vi "SP_OEE_2_test.vi"() -> ()   [LabVIEW 2017] (continued)
                      tunnel: w15923 -> [w16181]
                      tunnel: w15922 -> [w16177]
                      tunnel: [w16176] -> w15907
                      tunnel: w15921 -> [w16176]
                      tunnel: w15920 -> [w16237]
                      tunnel: w15919 -> [w16230]
                      tunnel: w15918 -> [w16221]
                      tunnel: w15917 -> [w16229]
                      tunnel: w15916 -> [w16219]
                      tunnel: w15915 -> [w16228]
                      tunnel: w15914 -> [w16217]
                      tunnel: w15913 -> [w16227]
                      tunnel: w15912 -> [w16215]
                      tunnel: w15911 -> [w16251]
                      tunnel: w15910 -> [w16250]
                      tunnel: w15909 -> [w16226]
                      tunnel: w15908 -> [w16213]
                      tunnel: [w16251] -> w15906
                      tunnel: [w16250] -> w15905
                      tunnel: [w16244] -> w15904
                      tunnel: [w16237] -> w15903
                      tunnel: [w16236] -> w15902
                      tunnel: [w16235] -> w15901
                      tunnel: [w16234] -> w15900
                      tunnel: [w16233] -> w15899
                      tunnel: [w16232] -> w15898
                      tunnel: [w16231] -> w15897
                      tunnel: [w16230] -> w15896
                      tunnel: [w16229] -> w15895
                      tunnel: [w16228] -> w15894
                      tunnel: [w16227] -> w15893
                      tunnel: [w16226] -> w15892
                      tunnel: [w16211] -> w15891
                      tunnel: w15907 -> [w16211]
                      tunnel: [w16264] -> _
                      tunnel: [w16260] -> _
                      tunnel: w15906 -> [w16261]
                      tunnel: w15905 -> [w16264]
                      tunnel: w15904 -> [w16255]
                      tunnel: w15903 -> [w16262]
                      tunnel: w15902 -> [_]
                      tunnel: w15901 -> [_]
                      tunnel: w15900 -> [_]
                      tunnel: w15899 -> [w16252]
                      tunnel: w15898 -> [_]
                      tunnel: w15897 -> [w16256]
                      tunnel: w15896 -> [_]
                      tunnel: w15895 -> [_]
                      tunnel: w15894 -> [_]
                      tunnel: w15893 -> [w16253]
                      tunnel: w15892 -> [_]
                      tunnel: w15891 -> [w16259]
                      frame #0 {
                        w15995 = "%Y-%m-%d" ("time format string (%c)")
                        n2900 = Decimal String To Number(string=w15981) -> (number=w15982:i32)  [unwired: 2 in, 1 out]
                        n2901 = property on="Table" class="Tbl (strict)"("Visible"=TRUE) -> ()  [unwired: 2 in, 2 out]
                        n2902 = Format Date/Time String(time format string (%c)=w15995, seconds (now)=w15987) -> (date/time string=w15996:string)  [unwired: 1 in]
                        n2903 = Format Date/Time String(time format string (%c)=w15995, seconds (now)=w15986) -> (date/time string=w15994:string)  [unwired: 1 in]
                        n2904 = Format Into String(format string="Where BREAKDOWN_DATE between '%s' and '%s' and  SHIFT_ID = '%d'  ", w15996, w15994, w15982) -> (resulting string=w15993:string)  [unwired: 2 in, 1 out]
                        n2905 = call <vilib>:"DB Tools Select Data.vi"("condition"=w15993, "error in (no error)"=w16002, "columns"=string[] ["BREAKDOWN_DATE"], "table"="STATION_1_LOG_HISTORY", "connection reference"=w16004) -> ("error out"=w15989:errorcluster, "data"=w15992:variant[][], "connection reference out"=w16003:T2)  [unwired: 1 in]
                        n2906 = property on="Table 2" class="Tbl (strict)"("Visible"=FALSE) -> ()  [unwired: 2 in, 2 out]
                        n2907 = xnode "Database Variant To Data"("database variant"=w15992, "error in (no error)"=w15989, "type"=string[][] [] ("Elements Found")) -> ("data"=w15990:string[][], "error out"=w15988:errorcluster)
                        n2908 = Index Array(array=w15990, index (col)=0 ("disabled index (col)")) -> (element=w15998:string[])  [unwired: 1 in]
                        n2909 = call "Search_1d_array_element.vi"("Count in"=string[] [] ("Elements Found"), "BD Date"=w15998, "Elements Found in"=string[] [] ("Elements Found")) -> ("Elements Found out"=w15985:string[])  [unwired: 4 in, 2 out]
                        n2910 = Build Array(w15985) -> (w16008:string[][])
                        n2911 = Transpose 2D Array(2D array=w16008) -> (transposed array=w16007:string[][])
                      }
                      frame #1 {
                        n2912 = disable-structure shown="Enabled" {
                          disable-tunnel: w16070 -> [w16081 w16083]
                          disable-tunnel: [w16080 w16083] -> w16069
                          disable-tunnel: w16068 -> [w16079 w16084]
                          disable-tunnel: [w16078 w16084] -> w16067
                          disable-tunnel: w16065 -> [w16076 _]
                          disable-tunnel: w16064 -> [w16075 _]
                          disable-tunnel: [w16074 _] -> w16063
                          disable-tunnel: [w16073 _] -> w16060
                          disable-tunnel: w16058 -> [w16072 _]
                          disable-tunnel: w16055 -> [w16071 w16082]
                          disable-tunnel: [_ w16082] -> w16054
                          frame Disabled {
                            n2913 = call "Stack_holderwise_total_bd_count_&_duration_2.vi"("Refnum in"=w16081, "BREAKDOWN_STK_HOLD_ID"=1, "condition"=w16072, "Form Date"=w16076, "To Date"=w16075, "error in (no error)"=w16079, "Shift"=w16071) -> ("Refnum out"=w16080:T2, "Count out"=w16074:string[], "appended array"=w16073:dbl[], "error out"=w16078:errorcluster)  [unwired: 5 in]
                          }
                          frame Enabled {
                          }
                        }
                        n2914 = call "NUMERIC TO STRING.vi"("appended array"=w16060) -> ("Array"=w16059:string[])  [unwired: 4 in]
                        n2915 = call "Insert_empty_element_with_zero.vi"("searched date"=w16063, "fixed date"=w16061) -> ("O/P"=w16056:string[])  [unwired: 9 in]
                        n2916 = call "Insert_empty_element_with_zero.vi"("searched date"=w16059, "fixed date"=w16061) -> ("O/P"=w16062:string[])  [unwired: 9 in]
                      }
                      frame #2 {
                        n2917 = disable-structure shown="Enabled" {
                          disable-tunnel: w16100 -> [w16114 w16116]
                          disable-tunnel: [w16113 w16116] -> w16099
                          disable-tunnel: w16098 -> [w16112 w16117]
                          disable-tunnel: [w16111 w16117] -> w16097
                          disable-tunnel: w16096 -> [w16110 _]
                          disable-tunnel: w16095 -> [w16109 _]
                          disable-tunnel: [w16108 _] -> w16094
                          disable-tunnel: [w16107 _] -> w16090
                          disable-tunnel: w16088 -> [w16106 _]
                          disable-tunnel: w16086 -> [w16104 w16115]
                          disable-tunnel: [_ w16115] -> w16085
                          frame Disabled {
                            n2918 = call "Stack_holderwise_total_bd_count_&_duration_2.vi"("Refnum in"=w16112, "BREAKDOWN_STK_HOLD_ID"=2, "condition"=w16106, "Form Date"=w16110, "To Date"=w16109, "error in (no error)"=w16114, "Shift"=w16104) -> ("Refnum out"=w16111:T2, "Count out"=w16108:string[], "appended array"=w16107:dbl[], "error out"=w16113:errorcluster)  [unwired: 5 in]
                          }
                          frame Enabled {
                          }
                        }
                        n2919 = call "Insert_empty_element_with_zero.vi"("searched date"=w16094, "fixed date"=w16091) -> ("O/P"=w16093:string[])  [unwired: 9 in]
                        n2920 = call "NUMERIC TO STRING.vi"("appended array"=w16090) -> ("Array"=w16089:string[])  [unwired: 4 in]
                        n2921 = call "Insert_empty_element_with_zero.vi"("searched date"=w16089, "fixed date"=w16091) -> ("O/P"=w16092:string[])  [unwired: 9 in]
                      }
                      frame #3 {
                        n2922 = disable-structure shown="Enabled" {
                          disable-tunnel: w16133 -> [w16149 w16151]
                          disable-tunnel: [w16148 w16151] -> w16132
                          disable-tunnel: w16131 -> [w16147 w16152]
                          disable-tunnel: [w16146 w16152] -> w16130
                          disable-tunnel: w16129 -> [w16145 _]
                          disable-tunnel: w16128 -> [w16144 _]
                          disable-tunnel: [w16143 _] -> w16127
                          disable-tunnel: [w16142 _] -> w16123
                          disable-tunnel: w16121 -> [w16141 _]
                          disable-tunnel: w16119 -> [w16139 w16150]
                          disable-tunnel: [_ w16150] -> w16118
                          frame Disabled {
                            n2923 = call "Stack_holderwise_total_bd_count_&_duration_2.vi"("Refnum in"=w16147, "BREAKDOWN_STK_HOLD_ID"=3, "condition"=w16141, "Form Date"=w16145, "To Date"=w16144, "error in (no error)"=w16149, "Shift"=w16139) -> ("Refnum out"=w16146:T2, "Count out"=w16143:string[], "appended array"=w16142:dbl[], "error out"=w16148:errorcluster)  [unwired: 5 in]
                          }
                          frame Enabled {
                          }
                        }
                        n2924 = call "Insert_empty_element_with_zero.vi"("searched date"=w16127, "fixed date"=w16124) -> ("O/P"=w16126:string[])  [unwired: 9 in]
                        n2925 = call "NUMERIC TO STRING.vi"("appended array"=w16123) -> ("Array"=w16122:string[])  [unwired: 4 in]
                        n2926 = call "Insert_empty_element_with_zero.vi"("searched date"=w16122, "fixed date"=w16124) -> ("O/P"=w16125:string[])  [unwired: 9 in]
                      }
                      frame #4 {
                        n2927 = call "Stack_holderwise_total_bd_count_&_duration_2.vi"("Refnum in"=w16167, "BREAKDOWN_STK_HOLD_ID"=4, "condition"=w16156, "Form Date"=w16164, "To Date"=w16163, "error in (no error)"=w16168, "Shift"=w16153) -> ("Refnum out"=w16166:T2, "Count out"=w16162:string[], "appended array"=w16158:dbl[], "error out"=w16165:errorcluster)  [unwired: 5 in]
                        n2928 = call "Insert_empty_element_with_zero.vi"("searched date"=w16162, "fixed date"=w16159) -> ("O/P"=w16161:string[])  [unwired: 9 in]
                        n2929 = call "NUMERIC TO STRING.vi"("appended array"=w16158) -> ("Array"=w16157:string[])  [unwired: 4 in]
                        n2930 = call "Insert_empty_element_with_zero.vi"("searched date"=w16157, "fixed date"=w16159) -> ("O/P"=w16160:string[])  [unwired: 9 in]
                      }
                      frame #5 {
                        n2931 = disable-structure shown="Enabled" {
                          disable-tunnel: w16189 -> [w16207 w16210]
                          disable-tunnel: [w16206 w16210] -> w16188
                          disable-tunnel: w16187 -> [w16205 w16209]
                          disable-tunnel: [w16204 w16209] -> w16186
                          disable-tunnel: w16185 -> [w16203 _]
                          disable-tunnel: w16184 -> [w16202 _]
                          disable-tunnel: [w16201 _] -> w16183
                          disable-tunnel: [w16200 _] -> w16179
                          disable-tunnel: w16177 -> [w16199 _]
                          frame Disabled {
                            n2932 = call "Stack_holderwise_total_bd_count_&_duration.vi"("Refnum in"=w16205, "BREAKDOWN_STK_HOLD_ID"=5, "condition"=w16199, "Form Date"=w16202, "To Date"=w16203, "error in (no error)"=w16207) -> ("Refnum out"=w16204:T2, "Count out"=w16201:string[], "appended array"=w16200:dbl[], "error out"=w16206:errorcluster)  [unwired: 6 in]
                          }
                          frame Enabled {
                          }
                        }
                        n2933 = call "NUMERIC TO STRING.vi"("appended array"=w16179) -> ("Array"=w16178:string[])  [unwired: 4 in]
                        n2934 = call "Insert_empty_element_with_zero.vi"("searched date"=w16183, "fixed date"=w16181) -> ("O/P"=w16182:string[])  [unwired: 9 in]
                        n2935 = call "Insert_empty_element_with_zero.vi"("searched date"=w16178, "fixed date"=w16181) -> ("O/P"=w16180:string[])  [unwired: 9 in]
                      }
                      frame #6 {
                        n2936 = call "String to numeric.vi"("Array"=w16221) -> ("Array 2"=w16220:dbl[])  [unwired: 4 in]
                        n2937 = call "String to numeric.vi"("Array"=w16219) -> ("Array 2"=w16218:dbl[])  [unwired: 4 in]
                        n2938 = call "String to numeric.vi"("Array"=w16217) -> ("Array 2"=w16216:dbl[])  [unwired: 4 in]
                        n2939 = call "String to numeric.vi"("Array"=w16215) -> ("Array 2"=w16214:dbl[])  [unwired: 4 in]
                        n2940 = call "String to numeric.vi"("Array"=w16213) -> ("Array 2"=w16212:dbl[])  [unwired: 4 in]
                        n2941 = Decimal String To Number(string=w16226) -> (number=w16245:i32[])  [unwired: 2 in, 1 out]
                        n2942 = Decimal String To Number(string=w16227) -> (number=w16246:i32[])  [unwired: 2 in, 1 out]
                        n2943 = Decimal String To Number(string=w16228) -> (number=w16247:i32[])  [unwired: 2 in, 1 out]
                        n2944 = Decimal String To Number(string=w16229) -> (number=w16248:i32[])  [unwired: 2 in, 1 out]
                        n2945 = Decimal String To Number(string=w16230) -> (number=w16243:i32[])  [unwired: 2 in, 1 out]
                        n2946 = Compound Arithmetic op=ADD(w16220, w16218, w16216, w16214, w16212) -> (w16223:dbl[])
                        n2947 = Build Array(w16221) -> (w16242:string[][])
                        n2948 = Build Array(w16219) -> (w16241:string[][])
                        n2949 = Build Array(w16217) -> (w16240:string[][])
                        n2950 = Build Array(w16215) -> (w16239:string[][])
                        n2951 = Build Array(w16213) -> (w16238:string[][])
                        n2952 = Number To Fractional String(number=w16223, precision (6)=i16 2) -> (F-format string=w16222:string[])  [unwired: 2 in]
                        n2953 = Compound Arithmetic op=ADD(w16245, w16246, w16247, w16248, w16243) -> (w16249:i32[])
                        n2954 = Transpose 2D Array(2D array=w16242) -> (transposed array=w16236:string[][])
                        n2955 = Transpose 2D Array(2D array=w16241) -> (transposed array=w16235:string[][])
                        n2956 = Transpose 2D Array(2D array=w16240) -> (transposed array=w16234:string[][])
                        n2957 = Transpose 2D Array(2D array=w16239) -> (transposed array=w16233:string[][])
                        n2958 = Transpose 2D Array(2D array=w16238) -> (transposed array=w16232:string[][])
                        n2959 = Number To Decimal String(number=w16249) -> (decimal integer string=w16244:string[])  [unwired: 1 in]
                        n2960 = Build Array(w16222) -> (w16225:string[][])
                        n2961 = Transpose 2D Array(2D array=w16225) -> (transposed array=w16231:string[][])
                      }
                      frame #7 {
                        w16254 = string[] [""]
                        n2962 = Insert Into Array(array=w16262, index (col)=1 ("disabled index (col)"), new element #1=w16254, new element #2=w16254, new element #3=w16254, new element #4=w16254, new element #5=w16254, new element #6=w16254, new element #7=w16253, new element #8=w16252, new element #9=w16254, new element #10=w16254, new element #11=w16255, new element #12=w16256) -> (w16258:string[][])  [unwired: 1 in]
                        n2963 = call "flot graph for month n year.vi"("BD Date"=w16259, "error in (no error)"=w16261, "Count total"=w16255) -> ("error out"=w16260:errorcluster, "Run-Time Status"=w16257:cluster{"Array 2":timestamp[], dbl[]})  [unwired: 7 in]
                        n2964 = local write "Run-Time Status"(w16257) -> ()
                        n2965 = local write "Table"(w16258) -> ()
                      }
                    }
                  }
                  frame "3" {
                    n2966 = flat-sequence {
                      tunnel: w16274 -> [w16388]
                      tunnel: w16273 -> [w16386]
                      tunnel: [w16372] -> w16364
                      tunnel: [w16387] -> w16363
                      tunnel: w16272 -> [_]
                      tunnel: [w16391] -> w16362
                      tunnel: [w16371] -> w16361
                      tunnel: [w16370] -> w16360
                      tunnel: [w16369] -> w16359
                      tunnel: w16271 -> [w16371]
                      tunnel: w16270 -> [w16370]
                      tunnel: ["Where BREAKDOWN_DATE between '%s'and '%s' and BREAKDOWN_STK_HOLD_ID ='%d' and  SHIFT_ID = '%d' "] -> w16358
                      tunnel: [w16369] -> w16357
                      tunnel: w16269 -> [w16365]
                      tunnel: [w16365] -> w16268
                      tunnel: w16364 -> [w16452]
                      tunnel: w16363 -> [w16454]
                      tunnel: w16362 -> [w16450]
                      tunnel: w16361 -> [w16449]
                      tunnel: w16360 -> [w16448]
                      tunnel: [w16451] -> w16356
                      tunnel: [w16453] -> w16355
                      tunnel: [w16450] -> w16354
                      tunnel: [w16440] -> w16353
                      tunnel: [w16446] -> w16352
                      tunnel: [w16449] -> w16351
                      tunnel: [w16448] -> w16350
                      tunnel: w16359 -> [w16445]
                      tunnel: [w16445] -> w16349
                      tunnel: w16358 -> [w16442]
                      tunnel: [w16442] -> w16348
                      tunnel: [w16441] -> w16347
                      tunnel: w16357 -> [w16441]
                      tunnel: w16268 -> [w16439]
                      tunnel: [w16438] -> w16267
                      tunnel: w16356 -> [w16484]
                      tunnel: w16355 -> [w16482]
                      tunnel: w16354 -> [w16487]
                      tunnel: w16353 -> [w16486]
                      tunnel: w16352 -> [w16485]
                      tunnel: w16351 -> [w16480]
                      tunnel: w16350 -> [w16479]
                      tunnel: [w16487] -> w16346
                      tunnel: [w16486] -> w16345
                      tunnel: [w16485] -> w16344
                      tunnel: [w16483] -> w16343
                      tunnel: [w16477] -> w16342
                      tunnel: [w16476] -> w16341
                      tunnel: [w16481] -> w16340
                      tunnel: [w16480] -> w16339
                      tunnel: [w16479] -> w16338
                      tunnel: w16349 -> [w16475]
                      tunnel: [w16475] -> w16337
                      tunnel: w16348 -> [w16472]
                      tunnel: [w16472] -> w16336
                      tunnel: [w16471] -> w16335
                      tunnel: w16347 -> [w16471]
                      tunnel: w16267 -> [w16470]
                      tunnel: [w16469] -> w16266
                      tunnel: w16346 -> [w16522]
                      tunnel: w16345 -> [w16521]
                      tunnel: w16344 -> [w16520]
                      tunnel: w16343 -> [w16517]
                      tunnel: w16342 -> [w16519]
                      tunnel: w16341 -> [w16518]
                      tunnel: w16340 -> [w16515]
                      tunnel: w16339 -> [w16513]
                      tunnel: w16338 -> [w16512]
                      tunnel: [w16522] -> w16334
                      tunnel: [w16521] -> w16333
                      tunnel: [w16520] -> w16332
                      tunnel: [w16519] -> w16331
                      tunnel: [w16518] -> w16330
                      tunnel: [w16516] -> w16329
                      tunnel: [w16510] -> w16328
                      tunnel: [w16509] -> w16327
                      tunnel: [w16514] -> w16326
                      tunnel: [w16513] -> w16325
                      tunnel: [w16512] -> w16324
                      tunnel: w16337 -> [w16508]
                      tunnel: [w16508] -> w16323
                      tunnel: w16336 -> [w16505]
                      tunnel: [w16505] -> w16322
                      tunnel: [w16504] -> w16321
                      tunnel: w16335 -> [w16504]
                      tunnel: w16266 -> [w16503]
                      tunnel: [w16502] -> w16265
                      tunnel: w16334 -> [w16559]
                      tunnel: w16333 -> [w16558]
                      tunnel: w16332 -> [w16557]
                      tunnel: w16331 -> [w16556]
                      tunnel: w16330 -> [w16555]
                      tunnel: w16329 -> [w16552]
                      tunnel: w16328 -> [w16554]
                      tunnel: w16327 -> [w16553]
                      tunnel: w16326 -> [w16551]
                      tunnel: w16325 -> [w16548]
                      tunnel: w16324 -> [w16547]
                      tunnel: [w16559] -> w16320
                      tunnel: [w16558] -> w16319
                      tunnel: [w16557] -> w16318
                      tunnel: [w16556] -> w16317
                      tunnel: [w16555] -> w16316
                      tunnel: [w16554] -> w16315
                      tunnel: [w16553] -> w16314
                      tunnel: [w16550] -> w16313
                      tunnel: [w16549] -> w16312
                      tunnel: [w16545] -> w16311
                      tunnel: [w16544] -> w16310
                      tunnel: [w16548] -> w16309
                      tunnel: [w16547] -> w16308
                      tunnel: w16323 -> [w16543]
                      tunnel: [w16543] -> w16307
                      tunnel: w16322 -> [w16540]
                      tunnel: [w16540] -> w16306
                      tunnel: [w16539] -> w16305
                      tunnel: w16321 -> [w16539]
                      tunnel: w16265 -> [w16537]
                      tunnel: w16320 -> [w16582]
                      tunnel: w16319 -> [w16581]
                      tunnel: w16318 -> [w16580]
                      tunnel: w16317 -> [w16579]
                      tunnel: w16316 -> [w16578]
                      tunnel: w16315 -> [w16577]
                      tunnel: w16314 -> [w16576]
                      tunnel: w16313 -> [w16571]
                      tunnel: w16312 -> [w16573]
                      tunnel: w16311 -> [w16575]
                      tunnel: w16310 -> [w16574]
                      tunnel: w16309 -> [w16568]
                      tunnel: w16308 -> [w16569]
                      tunnel: [w16582] -> w16304
                      tunnel: [w16581] -> w16303
                      tunnel: [w16580] -> w16302
                      tunnel: [w16579] -> w16301
                      tunnel: [w16578] -> w16300
                      tunnel: [w16577] -> w16299
                      tunnel: [w16576] -> w16298
                      tunnel: [w16575] -> w16297
                      tunnel: [w16574] -> w16296
                      tunnel: [w16572] -> w16295
                      tunnel: [w16570] -> w16294
                      tunnel: [w16566] -> w16293
                      tunnel: [w16564] -> w16292
                      tunnel: w16307 -> [w16565]
                      tunnel: w16306 -> [w16561]
                      tunnel: [w16560] -> w16291
                      tunnel: w16305 -> [w16560]
                      tunnel: w16304 -> [w16621]
                      tunnel: w16303 -> [w16614]
                      tunnel: w16302 -> [w16605]
                      tunnel: w16301 -> [w16613]
                      tunnel: w16300 -> [w16603]
                      tunnel: w16299 -> [w16612]
                      tunnel: w16298 -> [w16601]
                      tunnel: w16297 -> [w16611]
                      tunnel: w16296 -> [w16599]
                      tunnel: w16295 -> [w16635]
                      tunnel: w16294 -> [w16634]
                      tunnel: w16293 -> [w16610]
                      tunnel: w16292 -> [w16597]
                      tunnel: [w16635] -> w16290
                      tunnel: [w16634] -> w16289
                      tunnel: [w16628] -> w16288
                      tunnel: [w16621] -> w16287
                      tunnel: [w16620] -> w16286
                      tunnel: [w16619] -> w16285
                      tunnel: [w16618] -> w16284
                      tunnel: [w16617] -> w16283
                      tunnel: [w16616] -> w16282
                      tunnel: [w16615] -> w16281
                      tunnel: [w16614] -> w16280
                      tunnel: [w16613] -> w16279
                      tunnel: [w16612] -> w16278
                      tunnel: [w16611] -> w16277
                      tunnel: [w16610] -> w16276
                      tunnel: [w16595] -> w16275
                      tunnel: w16291 -> [w16595]
                      tunnel: [w16648] -> _
                      tunnel: [w16644] -> _
                      tunnel: w16290 -> [w16645]
                      tunnel: w16289 -> [w16648]
                      tunnel: w16288 -> [w16639]
                      tunnel: w16287 -> [w16646]
                      tunnel: w16286 -> [_]
                      tunnel: w16285 -> [_]
                      tunnel: w16284 -> [_]
                      tunnel: w16283 -> [w16636]
                      tunnel: w16282 -> [_]
                      tunnel: w16281 -> [w16640]
                      tunnel: w16280 -> [_]
                      tunnel: w16279 -> [_]
                      tunnel: w16278 -> [_]
                      tunnel: w16277 -> [w16637]
                      tunnel: w16276 -> [_]
                      tunnel: w16275 -> [w16643]
                      frame #0 {
                        w16379 = "%Y-%m-%d" ("time format string (%c)")
                        n2967 = Decimal String To Number(string=w16365) -> (number=w16366:i32)  [unwired: 2 in, 1 out]
                        n2968 = property on="Table" class="Tbl (strict)"("Visible"=TRUE) -> ()  [unwired: 2 in, 2 out]
                        n2969 = Format Date/Time String(time format string (%c)=w16379, seconds (now)=w16371) -> (date/time string=w16380:string)  [unwired: 1 in]
                        n2970 = Format Date/Time String(time format string (%c)=w16379, seconds (now)=w16370) -> (date/time string=w16378:string)  [unwired: 1 in]
                        n2971 = Format Into String(format string="Where BREAKDOWN_DATE between '%s' and '%s' and  SHIFT_ID = '%d'  ", w16380, w16378, w16366) -> (resulting string=w16377:string)  [unwired: 2 in, 1 out]
                        n2972 = call <vilib>:"DB Tools Select Data.vi"("condition"=w16377, "error in (no error)"=w16386, "columns"=string[] ["BREAKDOWN_DATE"], "table"="STATION_1_LOG_HISTORY", "connection reference"=w16388) -> ("error out"=w16373:errorcluster, "data"=w16376:variant[][], "connection reference out"=w16387:T2)  [unwired: 1 in]
                        n2973 = property on="Table 2" class="Tbl (strict)"("Visible"=FALSE) -> ()  [unwired: 2 in, 2 out]
                        n2974 = xnode "Database Variant To Data"("database variant"=w16376, "error in (no error)"=w16373, "type"=string[][] [] ("Elements Found")) -> ("data"=w16374:string[][], "error out"=w16372:errorcluster)
                        n2975 = Index Array(array=w16374, index (col)=0 ("disabled index (col)")) -> (element=w16382:string[])  [unwired: 1 in]
                        n2976 = call "Search_1d_array_element.vi"("Count in"=string[] [] ("Elements Found"), "BD Date"=w16382, "Elements Found in"=string[] [] ("Elements Found")) -> ("Elements Found out"=w16369:string[])  [unwired: 4 in, 2 out]
                        n2977 = Build Array(w16369) -> (w16392:string[][])
                        n2978 = Transpose 2D Array(2D array=w16392) -> (transposed array=w16391:string[][])
                      }
                      frame #1 {
                        n2979 = disable-structure shown="Enabled" {
                          disable-tunnel: w16454 -> [w16465 w16467]
                          disable-tunnel: [w16464 w16467] -> w16453
                          disable-tunnel: w16452 -> [w16463 w16468]
                          disable-tunnel: [w16462 w16468] -> w16451
                          disable-tunnel: w16449 -> [w16460 _]
                          disable-tunnel: w16448 -> [w16459 _]
                          disable-tunnel: [w16458 _] -> w16447
                          disable-tunnel: [w16457 _] -> w16444
                          disable-tunnel: w16442 -> [w16456 _]
                          disable-tunnel: w16439 -> [w16455 w16466]
                          disable-tunnel: [_ w16466] -> w16438
                          frame Disabled {
                            n2980 = call "Stack_holderwise_total_bd_count_&_duration_2.vi"("Refnum in"=w16465, "BREAKDOWN_STK_HOLD_ID"=1, "condition"=w16456, "Form Date"=w16460, "To Date"=w16459, "error in (no error)"=w16463, "Shift"=w16455) -> ("Refnum out"=w16464:T2, "Count out"=w16458:string[], "appended array"=w16457:dbl[], "error out"=w16462:errorcluster)  [unwired: 5 in]
                          }
                          frame Enabled {
                          }
                        }
                        n2981 = call "NUMERIC TO STRING.vi"("appended array"=w16444) -> ("Array"=w16443:string[])  [unwired: 4 in]
                        n2982 = call "Insert_empty_element_with_zero.vi"("searched date"=w16447, "fixed date"=w16445) -> ("O/P"=w16440:string[])  [unwired: 9 in]
                        n2983 = call "Insert_empty_element_with_zero.vi"("searched date"=w16443, "fixed date"=w16445) -> ("O/P"=w16446:string[])  [unwired: 9 in]
                      }
                      frame #2 {
                        n2984 = disable-structure shown="Enabled" {
                          disable-tunnel: w16484 -> [w16498 w16500]
                          disable-tunnel: [w16497 w16500] -> w16483
                          disable-tunnel: w16482 -> [w16496 w16501]
                          disable-tunnel: [w16495 w16501] -> w16481
                          disable-tunnel: w16480 -> [w16494 _]
                          disable-tunnel: w16479 -> [w16493 _]
                          disable-tunnel: [w16492 _] -> w16478
                          disable-tunnel: [w16491 _] -> w16474
                          disable-tunnel: w16472 -> [w16490 _]
                          disable-tunnel: w16470 -> [w16488 w16499]
                          disable-tunnel: [_ w16499] -> w16469
                          frame Disabled {
                            n2985 = call "Stack_holderwise_total_bd_count_&_duration_2.vi"("Refnum in"=w16496, "BREAKDOWN_STK_HOLD_ID"=2, "condition"=w16490, "Form Date"=w16494, "To Date"=w16493, "error in (no error)"=w16498, "Shift"=w16488) -> ("Refnum out"=w16495:T2, "Count out"=w16492:string[], "appended array"=w16491:dbl[], "error out"=w16497:errorcluster)  [unwired: 5 in]
                          }
                          frame Enabled {
                          }
                        }
                        n2986 = call "Insert_empty_element_with_zero.vi"("searched date"=w16478, "fixed date"=w16475) -> ("O/P"=w16477:string[])  [unwired: 9 in]
                        n2987 = call "NUMERIC TO STRING.vi"("appended array"=w16474) -> ("Array"=w16473:string[])  [unwired: 4 in]
                        n2988 = call "Insert_empty_element_with_zero.vi"("searched date"=w16473, "fixed date"=w16475) -> ("O/P"=w16476:string[])  [unwired: 9 in]
                      }
                      frame #3 {
                        n2989 = disable-structure shown="Enabled" {
                          disable-tunnel: w16517 -> [w16533 w16535]
                          disable-tunnel: [w16532 w16535] -> w16516
                          disable-tunnel: w16515 -> [w16531 w16536]
                          disable-tunnel: [w16530 w16536] -> w16514
                          disable-tunnel: w16513 -> [w16529 _]
                          disable-tunnel: w16512 -> [w16528 _]
                          disable-tunnel: [w16527 _] -> w16511
                          disable-tunnel: [w16526 _] -> w16507
                          disable-tunnel: w16505 -> [w16525 _]
                          disable-tunnel: w16503 -> [w16523 w16534]
                          disable-tunnel: [_ w16534] -> w16502
                          frame Disabled {
                            n2990 = call "Stack_holderwise_total_bd_count_&_duration_2.vi"("Refnum in"=w16531, "BREAKDOWN_STK_HOLD_ID"=3, "condition"=w16525, "Form Date"=w16529, "To Date"=w16528, "error in (no error)"=w16533, "Shift"=w16523) -> ("Refnum out"=w16530:T2, "Count out"=w16527:string[], "appended array"=w16526:dbl[], "error out"=w16532:errorcluster)  [unwired: 5 in]
                          }
                          frame Enabled {
                          }
                        }
                        n2991 = call "Insert_empty_element_with_zero.vi"("searched date"=w16511, "fixed date"=w16508) -> ("O/P"=w16510:string[])  [unwired: 9 in]
                        n2992 = call "NUMERIC TO STRING.vi"("appended array"=w16507) -> ("Array"=w16506:string[])  [unwired: 4 in]
                        n2993 = call "Insert_empty_element_with_zero.vi"("searched date"=w16506, "fixed date"=w16508) -> ("O/P"=w16509:string[])  [unwired: 9 in]
                      }
                      frame #4 {
                        n2994 = call "Stack_holderwise_total_bd_count_&_duration_2.vi"("Refnum in"=w16551, "BREAKDOWN_STK_HOLD_ID"=4, "condition"=w16540, "Form Date"=w16548, "To Date"=w16547, "error in (no error)"=w16552, "Shift"=w16537) -> ("Refnum out"=w16550:T2, "Count out"=w16546:string[], "appended array"=w16542:dbl[], "error out"=w16549:errorcluster)  [unwired: 5 in]
                        n2995 = call "Insert_empty_element_with_zero.vi"("searched date"=w16546, "fixed date"=w16543) -> ("O/P"=w16545:string[])  [unwired: 9 in]
                        n2996 = call "NUMERIC TO STRING.vi"("appended array"=w16542) -> ("Array"=w16541:string[])  [unwired: 4 in]
                        n2997 = call "Insert_empty_element_with_zero.vi"("searched date"=w16541, "fixed date"=w16543) -> ("O/P"=w16544:string[])  [unwired: 9 in]
                      }
                      frame #5 {
                        n2998 = disable-structure shown="Enabled" {
                          disable-tunnel: w16573 -> [w16591 w16594]
                          disable-tunnel: [w16590 w16594] -> w16572
                          disable-tunnel: w16571 -> [w16589 w16593]
                          disable-tunnel: [w16588 w16593] -> w16570
                          disable-tunnel: w16569 -> [w16587 _]
                          disable-tunnel: w16568 -> [w16586 _]
                          disable-tunnel: [w16585 _] -> w16567
                          disable-tunnel: [w16584 _] -> w16563
                          disable-tunnel: w16561 -> [w16583 _]
                          frame Disabled {
                            n2999 = call "Stack_holderwise_total_bd_count_&_duration.vi"("Refnum in"=w16589, "BREAKDOWN_STK_HOLD_ID"=5, "condition"=w16583, "Form Date"=w16586, "To Date"=w16587, "error in (no error)"=w16591) -> ("Refnum out"=w16588:T2, "Count out"=w16585:string[], "appended array"=w16584:dbl[], "error out"=w16590:errorcluster)  [unwired: 6 in]
                          }
                          frame Enabled {
                          }
                        }
                        n3000 = call "NUMERIC TO STRING.vi"("appended array"=w16563) -> ("Array"=w16562:string[])  [unwired: 4 in]
                        n3001 = call "Insert_empty_element_with_zero.vi"("searched date"=w16567, "fixed date"=w16565) -> ("O/P"=w16566:string[])  [unwired: 9 in]
                        n3002 = call "Insert_empty_element_with_zero.vi"("searched date"=w16562, "fixed date"=w16565) -> ("O/P"=w16564:string[])  [unwired: 9 in]
                      }
                      frame #6 {
                        n3003 = call "String to numeric.vi"("Array"=w16605) -> ("Array 2"=w16604:dbl[])  [unwired: 4 in]
                        n3004 = call "String to numeric.vi"("Array"=w16603) -> ("Array 2"=w16602:dbl[])  [unwired: 4 in]
                        n3005 = call "String to numeric.vi"("Array"=w16601) -> ("Array 2"=w16600:dbl[])  [unwired: 4 in]
                        n3006 = call "String to numeric.vi"("Array"=w16599) -> ("Array 2"=w16598:dbl[])  [unwired: 4 in]
                        n3007 = call "String to numeric.vi"("Array"=w16597) -> ("Array 2"=w16596:dbl[])  [unwired: 4 in]
                        n3008 = Decimal String To Number(string=w16610) -> (number=w16629:i32[])  [unwired: 2 in, 1 out]
                        n3009 = Decimal String To Number(string=w16611) -> (number=w16630:i32[])  [unwired: 2 in, 1 out]
                        n3010 = Decimal String To Number(string=w16612) -> (number=w16631:i32[])  [unwired: 2 in, 1 out]
                        n3011 = Decimal String To Number(string=w16613) -> (number=w16632:i32[])  [unwired: 2 in, 1 out]
                        n3012 = Decimal String To Number(string=w16614) -> (number=w16627:i32[])  [unwired: 2 in, 1 out]
                        n3013 = Compound Arithmetic op=ADD(w16604, w16602, w16600, w16598, w16596) -> (w16607:dbl[])
                        n3014 = Build Array(w16605) -> (w16626:string[][])
                        n3015 = Build Array(w16603) -> (w16625:string[][])
                        n3016 = Build Array(w16601) -> (w16624:string[][])
                        n3017 = Build Array(w16599) -> (w16623:string[][])
                        n3018 = Build Array(w16597) -> (w16622:string[][])
                        n3019 = Number To Fractional String(number=w16607, precision (6)=i16 2) -> (F-format string=w16606:string[])  [unwired: 2 in]
                        n3020 = Compound Arithmetic op=ADD(w16629, w16630, w16631, w16632, w16627) -> (w16633:i32[])
                        n3021 = Transpose 2D Array(2D array=w16626) -> (transposed array=w16620:string[][])
                        n3022 = Transpose 2D Array(2D array=w16625) -> (transposed array=w16619:string[][])
                        n3023 = Transpose 2D Array(2D array=w16624) -> (transposed array=w16618:string[][])
                        n3024 = Transpose 2D Array(2D array=w16623) -> (transposed array=w16617:string[][])
                        n3025 = Transpose 2D Array(2D array=w16622) -> (transposed array=w16616:string[][])
                        n3026 = Number To Decimal String(number=w16633) -> (decimal integer string=w16628:string[])  [unwired: 1 in]
                        n3027 = Build Array(w16606) -> (w16609:string[][])
                        n3028 = Transpose 2D Array(2D array=w16609) -> (transposed array=w16615:string[][])
                      }
                      frame #7 {
                        w16638 = string[] [""]
                        n3029 = Insert Into Array(array=w16646, index (col)=1 ("disabled index (col)"), new element #1=w16638, new element #2=w16638, new element #3=w16638, new element #4=w16638, new element #5=w16638, new element #6=w16638, new element #7=w16637, new element #8=w16636, new element #9=w16638, new element #10=w16638, new element #11=w16639, new element #12=w16640) -> (w16642:string[][])  [unwired: 1 in]
                        n3030 = call "flot graph for month n year.vi"("BD Date"=w16643, "error in (no error)"=w16645, "Count total"=w16639) -> ("error out"=w16644:errorcluster, "Run-Time Status"=w16641:cluster{"Array 2":timestamp[], dbl[]})  [unwired: 7 in]
                        n3031 = local write "Run-Time Status"(w16641) -> ()
                        n3032 = local write "Table"(w16642) -> ()
                      }
                    }
                  }
                  frame "all" {
                  }
                }
              }
              frame "Production" {
                n3033 = local read "Shift"() -> (w16649:string)
                n3034 = case shown="\"1\"" w16649 {
                  selector: w16649 -> [_ w17024 w17413 w17802 _]
                  tunnel: w16654 -> [w16659 w17029 w17418 w17807 _]
                  tunnel: w16653 -> [w16658 w17028 w17417 w17806 _]
                  tunnel: w16652 -> [w16657 w17027 w17416 w17805 _]
                  tunnel: w16651 -> [w16656 w17026 w17415 w17804 _]
                  tunnel: w16650 -> [w16655 w17025 w17414 w17803 _]
                  frame "ALL", Default {
                    n3035 = flat-sequence {
                      tunnel: w16659 -> [w16771]
                      tunnel: w16658 -> [w16769]
                      tunnel: [w16755] -> w16749
                      tunnel: [w16770] -> w16748
                      tunnel: w16657 -> [_]
                      tunnel: [w16774] -> w16747
                      tunnel: [w16754] -> w16746
                      tunnel: [w16753] -> w16745
                      tunnel: [w16751] -> w16744
                      tunnel: w16656 -> [w16754]
                      tunnel: w16655 -> [w16753]
                      tunnel: ["Where BREAKDOWN_DATE between '%s'and '%s' and BREAKDOWN_STK_HOLD_ID ='%d'  "] -> w16743
                      tunnel: [w16751] -> w16742
                      tunnel: w16749 -> [w16833]
                      tunnel: w16748 -> [w16835]
                      tunnel: w16747 -> [w16831]
                      tunnel: w16746 -> [w16830]
                      tunnel: w16745 -> [w16829]
                      tunnel: [w16832] -> w16741
                      tunnel: [w16834] -> w16740
                      tunnel: [w16831] -> w16739
                      tunnel: [w16821] -> w16738
                      tunnel: [w16827] -> w16737
                      tunnel: [w16830] -> w16736
                      tunnel: [w16829] -> w16735
                      tunnel: w16744 -> [w16826]
                      tunnel: [w16826] -> w16734
                      tunnel: w16743 -> [w16823]
                      tunnel: [w16823] -> w16733
                      tunnel: [w16822] -> w16732
                      tunnel: w16742 -> [w16822]
                      tunnel: w16741 -> [w16861]
                      tunnel: w16740 -> [w16859]
                      tunnel: w16739 -> [w16864]
                      tunnel: w16738 -> [w16863]
                      tunnel: w16737 -> [w16862]
                      tunnel: w16736 -> [w16857]
                      tunnel: w16735 -> [w16856]
                      tunnel: [w16864] -> w16731
                      tunnel: [w16863] -> w16730
                      tunnel: [w16862] -> w16729
                      tunnel: [w16860] -> w16728
                      tunnel: [w16854] -> w16727
                      tunnel: [w16853] -> w16726
                      tunnel: [w16858] -> w16725
                      tunnel: [w16857] -> w16724
                      tunnel: [w16856] -> w16723
                      tunnel: w16734 -> [w16852]
                      tunnel: [w16852] -> w16722
                      tunnel: w16733 -> [w16849]
                      tunnel: [w16849] -> w16721
                      tunnel: [w16848] -> w16720
                      tunnel: w16732 -> [w16848]
                      tunnel: w16731 -> [w16895]
                      tunnel: w16730 -> [w16894]
                      tunnel: w16729 -> [w16893]
                      tunnel: w16728 -> [w16890]
                      tunnel: w16727 -> [w16892]
                      tunnel: w16726 -> [w16891]
                      tunnel: w16725 -> [w16888]
                      tunnel: w16724 -> [w16886]
                      tunnel: w16723 -> [w16885]
                      tunnel: [w16895] -> w16719
                      tunnel: [w16894] -> w16718
                      tunnel: [w16893] -> w16717
                      tunnel: [w16892] -> w16716
                      tunnel: [w16891] -> w16715
                      tunnel: [w16889] -> w16714
                      tunnel: [w16883] -> w16713
                      tunnel: [w16882] -> w16712
                      tunnel: [w16887] -> w16711
                      tunnel: [w16886] -> w16710
                      tunnel: [w16885] -> w16709
                      tunnel: w16722 -> [w16881]
                      tunnel: [w16881] -> w16708
                      tunnel: w16721 -> [w16878]
                      tunnel: [w16878] -> w16707
                      tunnel: [w16877] -> w16706
                      tunnel: w16720 -> [w16877]
                      tunnel: w16719 -> [w16928]
                      tunnel: w16718 -> [w16927]
                      tunnel: w16717 -> [w16926]
                      tunnel: w16716 -> [w16925]
                      tunnel: w16715 -> [w16924]
                      tunnel: w16714 -> [w16921]
                      tunnel: w16713 -> [w16923]
                      tunnel: w16712 -> [w16922]
                      tunnel: w16711 -> [w16920]
                      tunnel: w16710 -> [w16917]
                      tunnel: w16709 -> [w16916]
                      tunnel: [w16928] -> w16705
                      tunnel: [w16927] -> w16704
                      tunnel: [w16926] -> w16703
                      tunnel: [w16925] -> w16702
                      tunnel: [w16924] -> w16701
                      tunnel: [w16923] -> w16700
                      tunnel: [w16922] -> w16699
                      tunnel: [w16919] -> w16698
                      tunnel: [w16918] -> w16697
                      tunnel: [w16914] -> w16696
                      tunnel: [w16913] -> w16695
                      tunnel: [w16917] -> w16694
                      tunnel: [w16916] -> w16693
                      tunnel: w16708 -> [w16912]
                      tunnel: [w16912] -> w16692
                      tunnel: w16707 -> [w16909]
                      tunnel: [w16909] -> w16691
                      tunnel: [w16908] -> w16690
                      tunnel: w16706 -> [w16908]
                      tunnel: w16705 -> [w16964]
                      tunnel: w16704 -> [w16963]
                      tunnel: w16703 -> [w16962]
                      tunnel: w16702 -> [w16961]
                      tunnel: w16701 -> [w16960]
                      tunnel: w16700 -> [w16959]
                      tunnel: w16699 -> [w16958]
                      tunnel: w16698 -> [w16953]
                      tunnel: w16697 -> [w16955]
                      tunnel: w16696 -> [w16957]
                      tunnel: w16695 -> [w16956]
                      tunnel: w16694 -> [w16950]
                      tunnel: w16693 -> [w16951]
                      tunnel: [w16964] -> w16689
                      tunnel: [w16963] -> w16688
                      tunnel: [w16962] -> w16687
                      tunnel: [w16961] -> w16686
                      tunnel: [w16960] -> w16685
                      tunnel: [w16959] -> w16684
                      tunnel: [w16958] -> w16683
                      tunnel: [w16957] -> w16682
                      tunnel: [w16956] -> w16681
                      tunnel: [w16954] -> w16680
                      tunnel: [w16952] -> w16679
                      tunnel: [w16948] -> w16678
                      tunnel: [w16946] -> w16677
                      tunnel: w16692 -> [w16947]
                      tunnel: w16691 -> [w16943]
                      tunnel: [w16942] -> w16676
                      tunnel: w16690 -> [w16942]
                      tunnel: w16689 -> [w16991]
                      tunnel: w16688 -> [w16984]
                      tunnel: w16687 -> [w16975]
                      tunnel: w16686 -> [w16983]
                      tunnel: w16685 -> [w16973]
                      tunnel: w16684 -> [w16982]
                      tunnel: w16683 -> [w16971]
                      tunnel: w16682 -> [w16981]
                      tunnel: w16681 -> [w16969]
                      tunnel: w16680 -> [w17005]
                      tunnel: w16679 -> [w17004]
                      tunnel: w16678 -> [w16980]
                      tunnel: w16677 -> [w16967]
                      tunnel: [w17005] -> w16675
                      tunnel: [w17004] -> w16674
                      tunnel: [w16998] -> w16673
                      tunnel: [w16991] -> w16672
                      tunnel: [w16990] -> w16671
                      tunnel: [w16989] -> w16670
                      tunnel: [w16988] -> w16669
                      tunnel: [w16987] -> w16668
                      tunnel: [w16986] -> w16667
                      tunnel: [w16985] -> w16666
                      tunnel: [w16984] -> w16665
                      tunnel: [w16983] -> w16664
                      tunnel: [w16982] -> w16663
                      tunnel: [w16981] -> w16662
                      tunnel: [w16980] -> w16661
                      tunnel: [w16965] -> w16660
                      tunnel: w16676 -> [w16965]
                      tunnel: [w17018] -> _
                      tunnel: [w17014] -> _
                      tunnel: w16675 -> [w17015]
                      tunnel: w16674 -> [w17018]
                      tunnel: w16673 -> [w17009]
                      tunnel: w16672 -> [w17016]
                      tunnel: w16671 -> [_]
                      tunnel: w16670 -> [_]
                      tunnel: w16669 -> [_]
                      tunnel: w16668 -> [_]
                      tunnel: w16667 -> [w17008]
                      tunnel: w16666 -> [w17010]
                      tunnel: w16665 -> [_]
                      tunnel: w16664 -> [_]
                      tunnel: w16663 -> [_]
                      tunnel: w16662 -> [_]
                      tunnel: w16661 -> [w17007]
                      tunnel: w16660 -> [w17013]
                      frame #0 {
                        w16762 = "%Y-%m-%d" ("time format string (%c)")
                        n3036 = property on="Table" class="Tbl (strict)"("Visible"=TRUE) -> ()  [unwired: 2 in, 2 out]
                        n3037 = Format Date/Time String(time format string (%c)=w16762, seconds (now)=w16754) -> (date/time string=w16763:string)  [unwired: 1 in]
                        n3038 = Format Date/Time String(time format string (%c)=w16762, seconds (now)=w16753) -> (date/time string=w16761:string)  [unwired: 1 in]
                        n3039 = Format Into String(format string="Where BREAKDOWN_DATE between '%s' and '%s' ", w16763, w16761) -> (resulting string=w16760:string)  [unwired: 2 in, 1 out]
                        n3040 = call <vilib>:"DB Tools Select Data.vi"("condition"=w16760, "error in (no error)"=w16769, "columns"=string[] ["BREAKDOWN_DATE"], "table"="STATION_1_LOG_HISTORY", "connection reference"=w16771) -> ("error out"=w16756:errorcluster, "data"=w16759:variant[][], "connection reference out"=w16770:T2)  [unwired: 1 in]
                        n3041 = property on="Table 2" class="Tbl (strict)"("Visible"=FALSE) -> ()  [unwired: 2 in, 2 out]
                        n3042 = xnode "Database Variant To Data"("database variant"=w16759, "error in (no error)"=w16756, "type"=string[][] [] ("Elements Found")) -> ("data"=w16757:string[][], "error out"=w16755:errorcluster)
                        n3043 = Index Array(array=w16757, index (col)=0 ("disabled index (col)")) -> (element=w16765:string[])  [unwired: 1 in]
                        n3044 = call "Search_1d_array_element.vi"("Count in"=string[] [] ("Elements Found"), "BD Date"=w16765, "Elements Found in"=string[] [] ("Elements Found")) -> ("Elements Found out"=w16751:string[])  [unwired: 4 in, 2 out]
                        n3045 = Build Array(w16751) -> (w16775:string[][])
                        n3046 = Transpose 2D Array(2D array=w16775) -> (transposed array=w16774:string[][])
                      }
                      frame #1 {
                        n3047 = disable-structure shown="Enabled" {
                          disable-tunnel: w16835 -> [w16845 w16846]
                          disable-tunnel: [w16844 w16846] -> w16834
                          disable-tunnel: w16833 -> [w16843 w16847]
                          disable-tunnel: [w16842 w16847] -> w16832
                          disable-tunnel: w16830 -> [w16840 _]
                          disable-tunnel: w16829 -> [w16839 _]
                          disable-tunnel: [w16838 _] -> w16828
                          disable-tunnel: [w16837 _] -> w16825
                          disable-tunnel: w16823 -> [w16836 _]
                          frame Disabled {
                            n3048 = call "Stack_holderwise_total_bd_count_&_duration.vi"("Refnum in"=w16845, "BREAKDOWN_STK_HOLD_ID"=1, "condition"=w16836, "Form Date"=w16840, "To Date"=w16839, "error in (no error)"=w16843) -> ("Refnum out"=w16844:T2, "Count out"=w16838:string[], "appended array"=w16837:dbl[], "error out"=w16842:errorcluster)  [unwired: 6 in]
                          }
                          frame Enabled {
                          }
                        }
                        n3049 = call "NUMERIC TO STRING.vi"("appended array"=w16825) -> ("Array"=w16824:string[])  [unwired: 4 in]
                        n3050 = call "Insert_empty_element_with_zero.vi"("searched date"=w16828, "fixed date"=w16826) -> ("O/P"=w16821:string[])  [unwired: 9 in]
                        n3051 = call "Insert_empty_element_with_zero.vi"("searched date"=w16824, "fixed date"=w16826) -> ("O/P"=w16827:string[])  [unwired: 9 in]
                      }
                      frame #2 {
                        n3052 = disable-structure shown="Enabled" {
                          disable-tunnel: w16861 -> [w16874 w16876]
                          disable-tunnel: [w16873 w16876] -> w16860
                          disable-tunnel: w16859 -> [w16872 w16875]
                          disable-tunnel: [w16871 w16875] -> w16858
                          disable-tunnel: w16857 -> [w16870 _]
                          disable-tunnel: w16856 -> [w16869 _]
                          disable-tunnel: [w16868 _] -> w16855
                          disable-tunnel: [w16867 _] -> w16851
                          disable-tunnel: w16849 -> [w16866 _]
                          frame Disabled {
                            n3053 = call "Stack_holderwise_total_bd_count_&_duration.vi"("Refnum in"=w16872, "BREAKDOWN_STK_HOLD_ID"=2, "condition"=w16866, "Form Date"=w16870, "To Date"=w16869, "error in (no error)"=w16874) -> ("Refnum out"=w16871:T2, "Count out"=w16868:string[], "appended array"=w16867:dbl[], "error out"=w16873:errorcluster)  [unwired: 6 in]
                          }
                          frame Enabled {
                          }
                        }
                        n3054 = call "Insert_empty_element_with_zero.vi"("searched date"=w16855, "fixed date"=w16852) -> ("O/P"=w16854:string[])  [unwired: 9 in]
                        n3055 = call "NUMERIC TO STRING.vi"("appended array"=w16851) -> ("Array"=w16850:string[])  [unwired: 4 in]
                        n3056 = call "Insert_empty_element_with_zero.vi"("searched date"=w16850, "fixed date"=w16852) -> ("O/P"=w16853:string[])  [unwired: 9 in]
                      }
                      frame #3 {
                        n3057 = disable-structure shown="Enabled" {
                          disable-tunnel: w16890 -> [w16905 w16907]
                          disable-tunnel: [w16904 w16907] -> w16889
                          disable-tunnel: w16888 -> [w16903 w16906]
                          disable-tunnel: [w16902 w16906] -> w16887
                          disable-tunnel: w16886 -> [w16901 _]
                          disable-tunnel: w16885 -> [w16900 _]
                          disable-tunnel: [w16899 _] -> w16884
                          disable-tunnel: [w16898 _] -> w16880
                          disable-tunnel: w16878 -> [w16897 _]
                          frame Disabled {
                            n3058 = call "Stack_holderwise_total_bd_count_&_duration.vi"("Refnum in"=w16903, "BREAKDOWN_STK_HOLD_ID"=3, "condition"=w16897, "Form Date"=w16901, "To Date"=w16900, "error in (no error)"=w16905) -> ("Refnum out"=w16902:T2, "Count out"=w16899:string[], "appended array"=w16898:dbl[], "error out"=w16904:errorcluster)  [unwired: 6 in]
                          }
                          frame Enabled {
                          }
                        }
                        n3059 = call "Insert_empty_element_with_zero.vi"("searched date"=w16884, "fixed date"=w16881) -> ("O/P"=w16883:string[])  [unwired: 9 in]
                        n3060 = call "NUMERIC TO STRING.vi"("appended array"=w16880) -> ("Array"=w16879:string[])  [unwired: 4 in]
                        n3061 = call "Insert_empty_element_with_zero.vi"("searched date"=w16879, "fixed date"=w16881) -> ("O/P"=w16882:string[])  [unwired: 9 in]
                      }
                      frame #4 {
                        n3062 = disable-structure shown="Enabled" {
                          disable-tunnel: w16921 -> [w16938 w16940]
                          disable-tunnel: w16920 -> [w16937 w16939]
                          disable-tunnel: [w16936 w16939] -> w16919
                          disable-tunnel: [w16935 w16940] -> w16918
                          disable-tunnel: w16917 -> [w16934 _]
                          disable-tunnel: w16916 -> [w16933 _]
                          disable-tunnel: [w16932 _] -> w16915
                          disable-tunnel: [w16931 _] -> w16911
                          disable-tunnel: w16909 -> [w16930 _]
                          frame Disabled {
                            n3063 = call "Stack_holderwise_total_bd_count_&_duration.vi"("Refnum in"=w16937, "BREAKDOWN_STK_HOLD_ID"=4, "condition"=w16930, "Form Date"=w16934, "To Date"=w16933, "error in (no error)"=w16938) -> ("Refnum out"=w16936:T2, "Count out"=w16932:string[], "appended array"=w16931:dbl[], "error out"=w16935:errorcluster)  [unwired: 6 in]
                          }
                          frame Enabled {
                          }
                        }
                        n3064 = call "Insert_empty_element_with_zero.vi"("searched date"=w16915, "fixed date"=w16912) -> ("O/P"=w16914:string[])  [unwired: 9 in]
                        n3065 = call "NUMERIC TO STRING.vi"("appended array"=w16911) -> ("Array"=w16910:string[])  [unwired: 4 in]
                        n3066 = call "Insert_empty_element_with_zero.vi"("searched date"=w16910, "fixed date"=w16912) -> ("O/P"=w16913:string[])  [unwired: 9 in]
                      }
                      frame #5 {
                        n3067 = call "Stack_holderwise_total_bd_count_&_duration.vi"("Refnum in"=w16953, "BREAKDOWN_STK_HOLD_ID"=5, "condition"=w16943, "Form Date"=w16950, "To Date"=w16951, "error in (no error)"=w16955) -> ("Refnum out"=w16952:T2, "Count out"=w16949:string[], "appended array"=w16945:dbl[], "error out"=w16954:errorcluster)  [unwired: 6 in]
                        n3068 = call "NUMERIC TO STRING.vi"("appended array"=w16945) -> ("Array"=w16944:string[])  [unwired: 4 in]
                        n3069 = call "Insert_empty_element_with_zero.vi"("searched date"=w16949, "fixed date"=w16947) -> ("O/P"=w16948:string[])  [unwired: 9 in]
                        n3070 = call "Insert_empty_element_with_zero.vi"("searched date"=w16944, "fixed date"=w16947) -> ("O/P"=w16946:string[])  [unwired: 9 in]
                      }
                      frame #6 {
                        n3071 = call "String to numeric.vi"("Array"=w16975) -> ("Array 2"=w16974:dbl[])  [unwired: 4 in]
                        n3072 = call "String to numeric.vi"("Array"=w16973) -> ("Array 2"=w16972:dbl[])  [unwired: 4 in]
                        n3073 = call "String to numeric.vi"("Array"=w16971) -> ("Array 2"=w16970:dbl[])  [unwired: 4 in]
                        n3074 = call "String to numeric.vi"("Array"=w16969) -> ("Array 2"=w16968:dbl[])  [unwired: 4 in]
                        n3075 = call "String to numeric.vi"("Array"=w16967) -> ("Array 2"=w16966:dbl[])  [unwired: 4 in]
                        n3076 = Decimal String To Number(string=w16980) -> (number=w16999:i32[])  [unwired: 2 in, 1 out]
                        n3077 = Decimal String To Number(string=w16981) -> (number=w17000:i32[])  [unwired: 2 in, 1 out]
                        n3078 = Decimal String To Number(string=w16982) -> (number=w17001:i32[])  [unwired: 2 in, 1 out]
                        n3079 = Decimal String To Number(string=w16983) -> (number=w17002:i32[])  [unwired: 2 in, 1 out]
                        n3080 = Decimal String To Number(string=w16984) -> (number=w16997:i32[])  [unwired: 2 in, 1 out]
                        n3081 = Compound Arithmetic op=ADD(w16974, w16972, w16970, w16968, w16966) -> (w16977:dbl[])
                        n3082 = Build Array(w16975) -> (w16996:string[][])
                        n3083 = Build Array(w16973) -> (w16995:string[][])
                        n3084 = Build Array(w16971) -> (w16994:string[][])
                        n3085 = Build Array(w16969) -> (w16993:string[][])
                        n3086 = Build Array(w16967) -> (w16992:string[][])
                        n3087 = Number To Fractional String(number=w16977, precision (6)=i16 2) -> (F-format string=w16976:string[])  [unwired: 2 in]
                        n3088 = Compound Arithmetic op=ADD(w16999, w17000, w17001, w17002, w16997) -> (w17003:i32[])
                        n3089 = Transpose 2D Array(2D array=w16996) -> (transposed array=w16990:string[][])
                        n3090 = Transpose 2D Array(2D array=w16995) -> (transposed array=w16989:string[][])
                        n3091 = Transpose 2D Array(2D array=w16994) -> (transposed array=w16988:string[][])
                        n3092 = Transpose 2D Array(2D array=w16993) -> (transposed array=w16987:string[][])
                        n3093 = Transpose 2D Array(2D array=w16992) -> (transposed array=w16986:string[][])
                        n3094 = Number To Decimal String(number=w17003) -> (decimal integer string=w16998:string[])  [unwired: 1 in]
                        n3095 = Build Array(w16976) -> (w16979:string[][])
                        n3096 = Transpose 2D Array(2D array=w16979) -> (transposed array=w16985:string[][])
                      }
                      frame #7 {
                        w17006 = string[] [""]
                        n3097 = Insert Into Array(array=w17016, index (col)=1 ("disabled index (col)"), new element #1=w17006, new element #2=w17006, new element #3=w17006, new element #4=w17006, new element #5=w17006, new element #6=w17006, new element #7=w17006, new element #8=w17006, new element #9=w17007, new element #10=w17008, new element #11=w17009, new element #12=w17010) -> (w17012:string[][])  [unwired: 1 in]
                        n3098 = call "flot graph for month n year.vi"("BD Date"=w17013, "error in (no error)"=w17015, "Count total"=w17009) -> ("error out"=w17014:errorcluster, "Run-Time Status"=w17011:cluster{"Array 2":timestamp[], dbl[]})  [unwired: 7 in]
                        n3099 = local write "Run-Time Status"(w17011) -> ()
                        n3100 = local write "Table"(w17012) -> ()
                      }
                    }
                  }
                  frame "3" {
                    n3101 = flat-sequence {
                      tunnel: w17029 -> [w17143]
                      tunnel: w17028 -> [w17141]
                      tunnel: [w17127] -> w17119
                      tunnel: [w17142] -> w17118
                      tunnel: w17027 -> [_]
                      tunnel: [w17146] -> w17117
                      tunnel: [w17126] -> w17116
                      tunnel: [w17125] -> w17115
                      tunnel: [w17124] -> w17114
                      tunnel: w17026 -> [w17126]
                      tunnel: w17025 -> [w17125]
                      tunnel: ["Where BREAKDOWN_DATE between '%s'and '%s' and BREAKDOWN_STK_HOLD_ID ='%d' and  SHIFT_ID = '%d' "] -> w17113
                      tunnel: [w17124] -> w17112
                      tunnel: w17024 -> [w17120]
                      tunnel: [w17120] -> w17023
                      tunnel: w17119 -> [w17207]
                      tunnel: w17118 -> [w17209]
                      tunnel: w17117 -> [w17205]
                      tunnel: w17116 -> [w17204]
                      tunnel: w17115 -> [w17203]
                      tunnel: [w17206] -> w17111
                      tunnel: [w17208] -> w17110
                      tunnel: [w17205] -> w17109
                      tunnel: [w17195] -> w17108
                      tunnel: [w17201] -> w17107
                      tunnel: [w17204] -> w17106
                      tunnel: [w17203] -> w17105
                      tunnel: w17114 -> [w17200]
                      tunnel: [w17200] -> w17104
                      tunnel: w17113 -> [w17197]
                      tunnel: [w17197] -> w17103
                      tunnel: [w17196] -> w17102
                      tunnel: w17112 -> [w17196]
                      tunnel: w17023 -> [w17194]
                      tunnel: [w17193] -> w17022
                      tunnel: w17111 -> [w17239]
                      tunnel: w17110 -> [w17237]
                      tunnel: w17109 -> [w17242]
                      tunnel: w17108 -> [w17241]
                      tunnel: w17107 -> [w17240]
                      tunnel: w17106 -> [w17235]
                      tunnel: w17105 -> [w17234]
                      tunnel: [w17242] -> w17101
                      tunnel: [w17241] -> w17100
                      tunnel: [w17240] -> w17099
                      tunnel: [w17238] -> w17098
                      tunnel: [w17232] -> w17097
                      tunnel: [w17231] -> w17096
                      tunnel: [w17236] -> w17095
                      tunnel: [w17235] -> w17094
                      tunnel: [w17234] -> w17093
                      tunnel: w17104 -> [w17230]
                      tunnel: [w17230] -> w17092
                      tunnel: w17103 -> [w17227]
                      tunnel: [w17227] -> w17091
                      tunnel: [w17226] -> w17090
                      tunnel: w17102 -> [w17226]
                      tunnel: w17022 -> [w17225]
                      tunnel: [w17224] -> w17021
                      tunnel: w17101 -> [w17277]
                      tunnel: w17100 -> [w17276]
                      tunnel: w17099 -> [w17275]
                      tunnel: w17098 -> [w17272]
                      tunnel: w17097 -> [w17274]
                      tunnel: w17096 -> [w17273]
                      tunnel: w17095 -> [w17270]
                      tunnel: w17094 -> [w17268]
                      tunnel: w17093 -> [w17267]
                      tunnel: [w17277] -> w17089
                      tunnel: [w17276] -> w17088
                      tunnel: [w17275] -> w17087
                      tunnel: [w17274] -> w17086
                      tunnel: [w17273] -> w17085
                      tunnel: [w17271] -> w17084
                      tunnel: [w17265] -> w17083
                      tunnel: [w17264] -> w17082
                      tunnel: [w17269] -> w17081
                      tunnel: [w17268] -> w17080
                      tunnel: [w17267] -> w17079
                      tunnel: w17092 -> [w17263]
                      tunnel: [w17263] -> w17078
                      tunnel: w17091 -> [w17260]
                      tunnel: [w17260] -> w17077
                      tunnel: [w17259] -> w17076
                      tunnel: w17090 -> [w17259]
                      tunnel: w17021 -> [w17258]
                      tunnel: [w17257] -> w17020
                      tunnel: w17089 -> [w17314]
                      tunnel: w17088 -> [w17313]
                      tunnel: w17087 -> [w17312]
                      tunnel: w17086 -> [w17311]
                      tunnel: w17085 -> [w17310]
                      tunnel: w17084 -> [w17307]
                      tunnel: w17083 -> [w17309]
                      tunnel: w17082 -> [w17308]
                      tunnel: w17081 -> [w17306]
                      tunnel: w17080 -> [w17303]
                      tunnel: w17079 -> [w17302]
                      tunnel: [w17314] -> w17075
                      tunnel: [w17313] -> w17074
                      tunnel: [w17312] -> w17073
                      tunnel: [w17311] -> w17072
                      tunnel: [w17310] -> w17071
                      tunnel: [w17309] -> w17070
                      tunnel: [w17308] -> w17069
                      tunnel: [w17305] -> w17068
                      tunnel: [w17304] -> w17067
                      tunnel: [w17300] -> w17066
                      tunnel: [w17299] -> w17065
                      tunnel: [w17303] -> w17064
                      tunnel: [w17302] -> w17063
                      tunnel: w17078 -> [w17298]
                      tunnel: [w17298] -> w17062
                      tunnel: w17077 -> [w17295]
                      tunnel: [w17295] -> w17061
                      tunnel: [w17294] -> w17060
                      tunnel: w17076 -> [w17294]
                      tunnel: w17020 -> [w17293]
                      tunnel: [w17292] -> w17019
                      tunnel: w17075 -> [w17353]
                      tunnel: w17074 -> [w17352]
                      tunnel: w17073 -> [w17351]
                      tunnel: w17072 -> [w17350]
                      tunnel: w17071 -> [w17349]
                      tunnel: w17070 -> [w17348]
                      tunnel: w17069 -> [w17347]
                      tunnel: w17068 -> [w17342]
                      tunnel: w17067 -> [w17344]
                      tunnel: w17066 -> [w17346]
                      tunnel: w17065 -> [w17345]
                      tunnel: w17064 -> [w17339]
                      tunnel: w17063 -> [w17340]
                      tunnel: [w17353] -> w17059
                      tunnel: [w17352] -> w17058
                      tunnel: [w17351] -> w17057
